vi "Ćw.1.vi"() -> ()   [LabVIEW 2015]
panel:
  out "Array":dbl[](array[numeric])
  in  "Numeric":i32
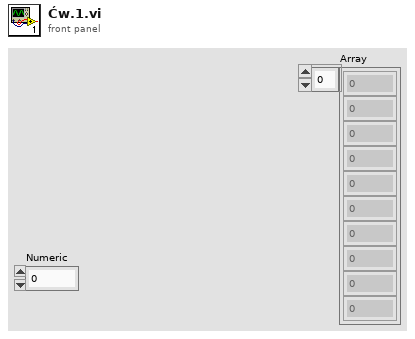
[diagram p1: front panel]
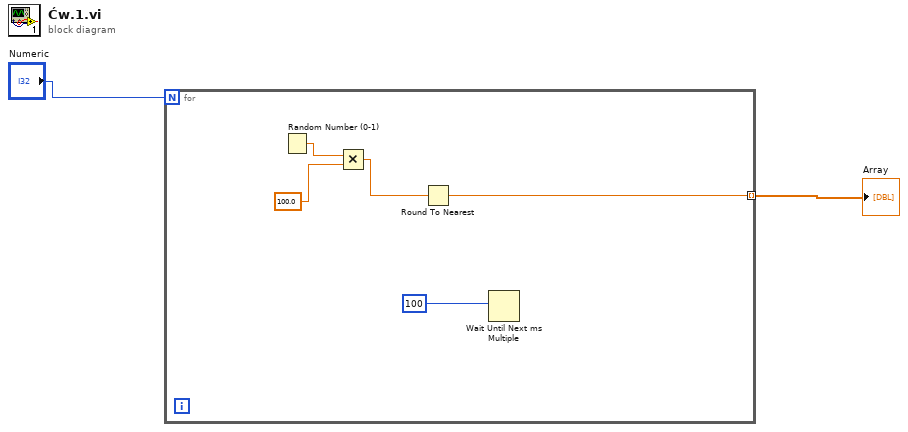
[diagram p0: block diagram]
diagram:
  n1 = for {
    N: "Numeric" -> [_]
    tunnel: [w4] -> w1 mode=indexing
    n2 = Random Number (0-1)() -> (number: 0 to 1=w7:dbl)
    n3 = Multiply(x=w7, y=100.0) -> (x*y=w5:dbl)
    n4 = Round To Nearest(number=w5) -> (nearest integer value=w4:dbl)
    n5 = Wait Until Next ms Multiple(millisecond multiple=u32 100 ("millisecond timer value")) -> ()  [unwired: 1 out]
  }
  "Array" <- w1
